vi "CfgWfrmMem.vi"(8 "error in (no error)":errorcluster, 11 "ScopePluginsBase in":refnum<class "ScopePluginsBase.lvclass">) -> (0 "error out":errorcluster, 3 "ScopePluginsBase out":refnum<class "ScopePluginsBase.lvclass">)   [LabVIEW 2018, in "ScopePlugins.lvlib" / "ScopePluginsBase.lvclass"]
uses:
  ScopePluginsBase.lvclass
  <userlib>/NIST/BaseClasses/Object_class/BaseObject.lvclass
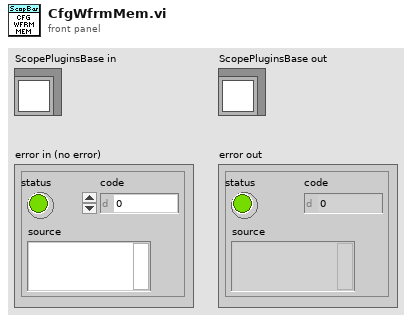
[diagram p1: front panel]
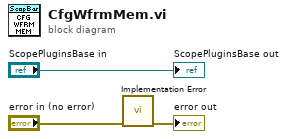
[diagram p0: block diagram]
diagram:
  n1 = call <userlib>:"Implementation Error.vi"("error in (no error)"="error in (no error)") -> ("error out"=→"error out":errorcluster)  [unwired: 10 in]
  "ScopePluginsBase out" <- "ScopePluginsBase in"
